vi "Read WiFi Config.vi"() -> (0 "error out":errorcluster)   [LabVIEW 2020]
panel:
  in  "Case Constant\n(See Context Help)":bool
  out "Default SSID":string
  out "Default SSID":string
  out "Current SSID":string
  out "Values (other)":dbl[](array[numeric]) format="%.2f"
  in  "Names (other)":string[](array[string])=["WIFI_STATUS", "WIFI_RSSI", "WIFI_DHCP_ENABLE_DEFAULT"]
  out "NumberToIP":string[](array[string])
  out "Error String":string
  out "ConnectionType Out":i32
  out "DeviceType Out":i32
  in  "Identifier":string="LJM_idANY"
  in  "ConnectionType":string="LJM_ctANY"
  in  "DeviceType":string="LJM_dtANY"
  out "Values (IP)":dbl[](array[numeric]) format="%.2f"
  in  "Names (IP)":string[](array[string])=["WIFI_IP", "WIFI_SUBNET", "WIFI_GATEWAY", "WIFI_IP_DEFAULT", "WIFI_SUBNET_DEFAULT", "WIFI_GATEWAY_DEFAULT"]
  # "// WiFi Status Codes:\n#define WIFI_ASSOCIATED                          2900\n#define WIFI_ASSOCIATING                        2901\n#define WIFI_ASSOCIATION_FAILED         2902\n#define WIFI_UNPOWERED                         2903\n#define WIFI_BOOTING_UP                         2904\n#define WIFI_COULD_NOT_START             2905\n#define WIFI_APPLYING_SETTINGS            2906\n#define WIFI_DHCP_STARTED                     2907\n#define WIFI_OTHER                                     2909"
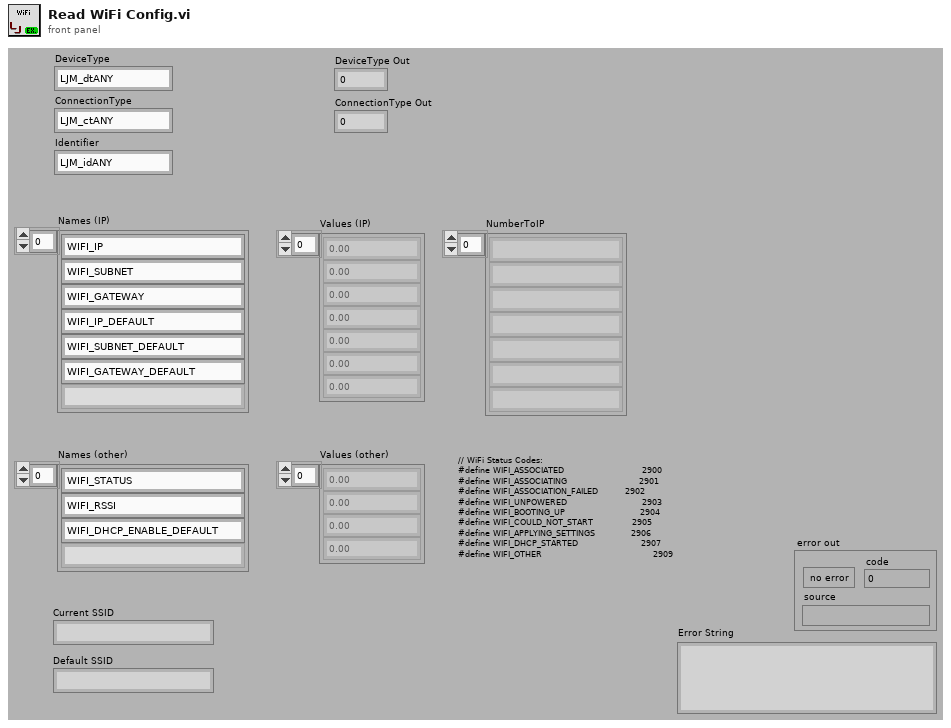
[diagram p1: front panel]
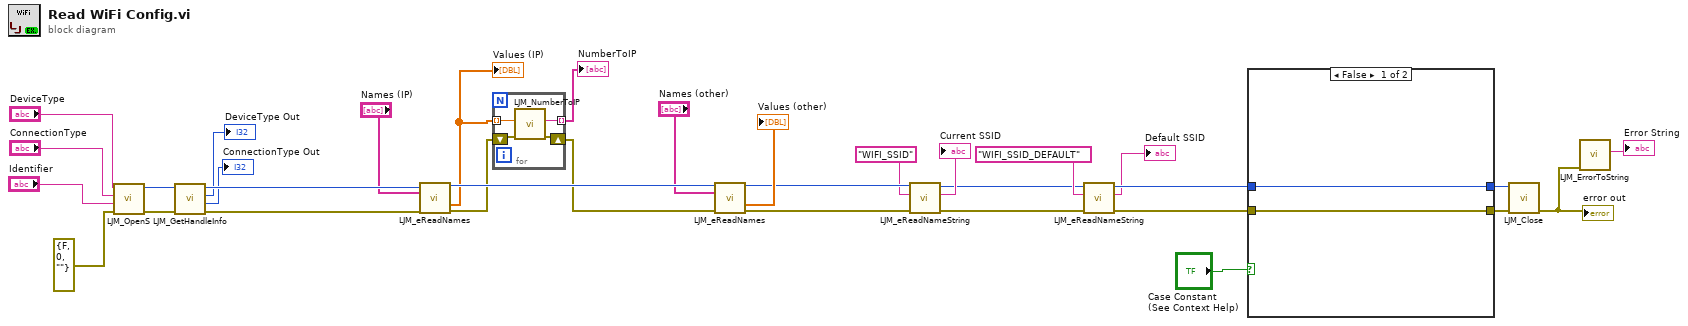
[diagram p0: block diagram]
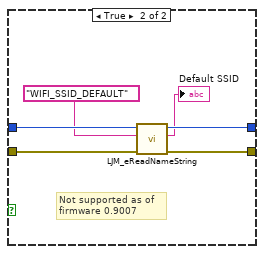
[diagram p2: hidden frame]
diagram:
  n1 = call "LJM_OpenS.vi"("error in"=errorcluster {"status"=FALSE, "code"=0, "source"=""} ("error in (no error)"), "Identifier"="Identifier", "ConnectionType"="ConnectionType", "DeviceType"="DeviceType") -> ("error out"=w32:errorcluster, "Handle"=w30:i32)  [unwired: 6 in]
  n2 = call "LJM_GetHandleInfo.vi"("error in"=w32, "Handle In"=w30) -> ("error out"=w31:errorcluster, "ConnectionType"=→"ConnectionType Out":i32, "DeviceType"=→"DeviceType Out":i32, "Handle Out"=w29:i32)  [unwired: 2 in, 4 out]
  n3 = call "LJM_eReadNames.vi"("Handle In"=w29, "aNames"="Names (IP)", "error in"=w31) -> ("Handle Out"=w20:i32, "aValuesOut"=w11:dbl[], "error out"=w9:errorcluster)  [unwired: 9 in, 1 out]
  "Values (IP)" <- w11
  n4 = for {
    tunnel: w11 -> [w37] mode=indexing
    tunnel: [w36] -> w10 mode=indexing
    shift-right: [w34] -> w8
    shift-left: w9 -> [w35]
    n5 = call "LJM_NumberToIP.vi"("error in"=w35, "Number"=w37) -> ("error out"=w34:errorcluster, "IPv4String"=w36:string)  [unwired: 8 in]
  }
  "NumberToIP" <- w10
  n6 = call "LJM_eReadNames.vi"("Handle In"=w20, "aNames"="Names (other)", "error in"=w8) -> ("Handle Out"=w17:i32, "aValuesOut"=→"Values (other)":dbl[], "error out"=w16:errorcluster)  [unwired: 9 in, 1 out]
  n7 = call "LJM_eReadNameString.vi"("error in"=w16, "Name"="WIFI_SSID", "Handle In"=w17) -> ("error out"=w4:errorcluster, "String"=→"Current SSID":string, "Handle Out"=w5:i32)  [unwired: 6 in]
  n8 = call "LJM_eReadNameString.vi"("error in"=w4, "Name"="WIFI_SSID_DEFAULT", "Handle In"=w5) -> ("error out"=w3:errorcluster, "String"=→"Default SSID":string, "Handle Out"=w2:i32)  [unwired: 6 in]
  n9 = case shown="False" "Case Constant\n(See Context Help)" {
    tunnel: w2 -> [w39 w45]
    tunnel: w3 -> [w38 w44]
    tunnel: [w38 w43] -> w13
    tunnel: [w39 w42] -> w12
    frame False {
    }
    frame True {
      # "Not supported as of\nfirmware 0.9007"
      n10 = call "LJM_eReadNameString.vi"("error in"=w44, "Name"="WIFI_SSID_DEFAULT", "Handle In"=w45) -> ("error out"=w43:errorcluster, "String"=→"Default SSID":string, "Handle Out"=w42:i32)  [unwired: 6 in]
    }
  }
  n11 = call "LJM_Close.vi"("error in"=w13, "Handle"=w12) -> ("error out"=w23:errorcluster)  [unwired: 9 in]
  "error out" <- w23
  n12 = call "LJM_ErrorToString.vi"("error in"=w23) -> ("String"=→"Error String":string)  [unwired: 10 in]
